vi "FileModifiedSinceCheck-Map.vi"(7 "mode":string(combo)="Check", 11 "file":path=path "") -> (1 "changed?":bool, 2 "unchanged?":bool)   [LabVIEW 2021]
panel:
  out "time(s)":dbl
  out "map":map{string, i32}(c390)
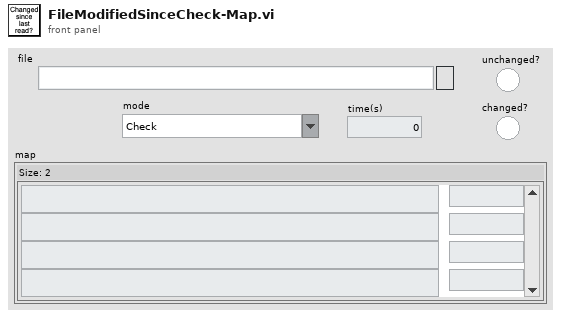
[diagram p1: front panel]
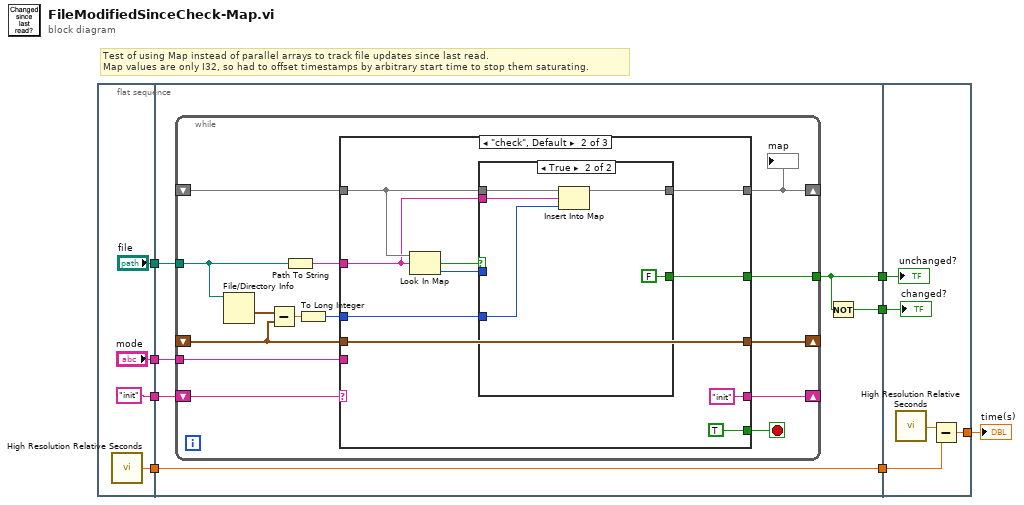
[diagram p0: block diagram]
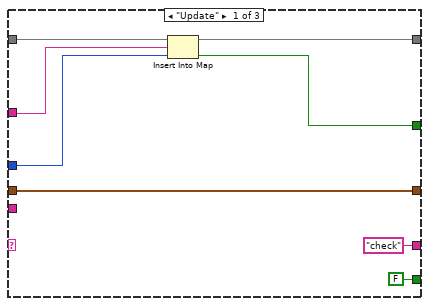
[diagram p2: hidden frame]
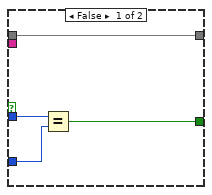
[diagram p3: hidden frame]
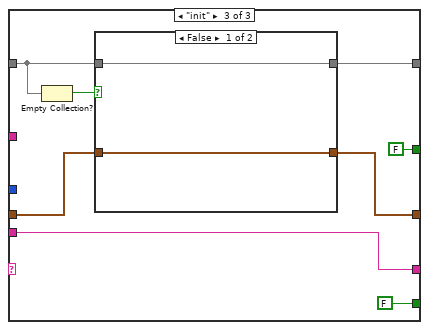
[diagram p4: hidden frame]
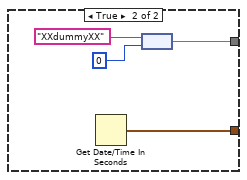
[diagram p5: hidden frame]
diagram:
  # "Test of using Map instead of parallel arrays to track file updates since last read.\nMap values are only I32, so had to offset timestamps by arbitrary start time to stop them saturating."
  n1 = flat-sequence {
    tunnel: ["mode"] -> w6
    tunnel: ["file"] -> w5
    tunnel: ["init"] -> w4
    tunnel: [w9] -> w2
    tunnel: [w18] -> w8
    tunnel: [w17] -> w7
    tunnel: w6 -> [w16]
    tunnel: w5 -> [w15]
    tunnel: w4 -> [w14]
    tunnel: [w13] -> w3
    tunnel: w2 -> [w13]
    tunnel: w8 -> [w77]
    tunnel: w7 -> [w78]
    tunnel: w3 -> [w75]
    tunnel: [w74] -> w1
    frame #0 {
      n2 = call <vilib>:"High Resolution Relative Seconds.vi"() -> ("relative seconds"=w9:dbl)
    }
    frame #1 {
      n3 = while {
        shift-right: [w31] -> _
        shift-left: _ -> [w32]
        shift-right: [w29] -> _
        shift-left: w14 -> [w30]
        tunnel: w15 -> [w22]
        tunnel: w16 -> [w27]
        shift-right: [w26] -> _
        shift-left: _ -> [w20]
        tunnel: [w19] -> w18
        stop <- w28 stop-if-true
        n4 = File/Directory Info(path=w22) -> (last mod=w24:timestamp)  [unwired: 1 in, 6 out]
        n5 = Subtract(x=w24, y=w20) -> (x-y=w23:dbl)
        n6 = Path To String(path=w22) -> (string=w25:string)
        n7 = To Long Integer(number=w23) -> (32bit integer=w21:i32)
        n8 = case shown="\"check\", Default" w30 {
          tunnel: w32 -> [w39 w49 w65]
          tunnel: [w38 w48 w67] -> w31
          tunnel: ["check" ("mode") "init" ("mode") w63] -> w29
          tunnel: [FALSE TRUE FALSE] -> w28
          tunnel: w27 -> [_ _ w63]
          tunnel: [w40 w45 w62] -> w26
          tunnel: w20 -> [w40 w45 w61]
          tunnel: w25 -> [w37 w44 _]
          tunnel: w21 -> [w36 w43 _]
          tunnel: [w35 w42 FALSE ("value unchanged?")] -> w19
          frame "Update" {
            n9 = Insert Into Map(map in=w39, key=w37, value=w36) -> (map out=w38:map{string, i32}, value unchanged?=w35:bool)  [unwired: 1 out]
          }
          frame "check", Default {
            n10 = Look In Map(map=w49, key=w44) -> (key not found?=w50:bool, value=w46:i32)  [unwired: 1 in]
            n11 = case shown="True" w50 {
              tunnel: w49 -> [w54 w59]
              tunnel: w44 -> [_ w58]
              tunnel: [w54 w57] -> w48
              tunnel: w43 -> [w52 w56]
              tunnel: w46 -> [w53 _]
              tunnel: [w51 FALSE] -> w42
              frame False {
                n12 = Equal?(x=w53, y=w52) -> (x = y?=w51:bool)
              }
              frame True {
                n13 = Insert Into Map(map in=w59, key=w58, value=w56) -> (map out=w57:map{string, i32})  [unwired: 2 out]
              }
            }
          }
          frame "init" {
            n14 = Empty Collection?(1:w65) -> (0:w66:bool)
            n15 = case shown="False" w66 {
              tunnel: [w69 w73] -> w67
              tunnel: w65 -> [w69 _]
              tunnel: [w68 w70] -> w62
              tunnel: w61 -> [w68 _]
              frame False {
              }
              frame True {
                n16 = Get Date/Time In Seconds() -> (seconds since 1Jan1904=w70:timestamp)
                n17 = node("XXdummyXX" ("key"), 0 ("value")) -> (w73:map{string, i32})
              }
            }
          }
        }
        "map" <- w31
      }
      n18 = Not(x=w18) -> (.not. x?=w17:bool)
    }
    frame #2 {
      n19 = call <vilib>:"High Resolution Relative Seconds.vi"() -> ("relative seconds"=w76:dbl)
      n20 = Subtract(x=w76, y=w75) -> (x-y=w74:dbl)
      "unchanged?" <- w77
      "changed?" <- w78
    }
  }
  "time(s)" <- w1
